vi "Dispense FN - OFF - Timer (SubVI).vi"(0 "Settings":T1={"ON Settings"={"Enable Dynamic Setpoint?"=TRUE, "Enable Dynamic Dispense Time?"=TRUE, "Enable Drain Rate Functions"=TRUE, "Dispense Sample Time (s)"=0.1, "Mass Average Samples"=20, "ON Timeout (sec)"=300.0, "1st Setpoint (% of Target)"=90.0, "2nd Setpoint (% of Target)"=95.0, "3rd Setpoint (% of Target)"=100.0, "Measure Dispense Delay (sec)"=10.0, "Minimum Spray Time (s)"=2.0, "Pump Reverse Time (s)"=10.0}, "OFF Settings"={"Drain Sample Time (s)"=0.1, "Drain Rate Ave Size"=100, "Drain Rate Limits (± g/sec)"=100.0, "Level Slope Range (± g/sec)"=0.05, "OFF Timeout (sec)"=300.0, "Near SP Slope Level (± g/sec)"=0.005, "Near Setpoint Threshold (%)"=99.0}, "Overshoot Settings"={"Time Limit (s)"=30.0, "Container MAX (g)"=1500.0, "Max FILL Slope (+/- g/sec)"=100.0, "% Overshot to Enable (>)"=3.0}, "FILL Timeout (s)"=300.0, "Full \nSettle Time (s)"=30.0, "Pre-Hydrate \nSpray Time (s)"=0.0, "Pre-Hydrate \nWait Time (s)"=10.0, "m Value "=1.0, "b Value"=0.0, "Enable Overshoot Adjust?"=FALSE} {"ON Settings"."Pump Reverse Time (s)" min=0.0 max=60.0; "OFF Settings"."Near SP Slope Level (± g/sec)" format="%.3g"; "OFF Settings"."Level Slope Range (± g/sec)" format="%.3g"}, 5 "Reset":bool) -> (14 "Sample":bool, 16 "Max Drain Complete?":bool, 19 "Elapsed Time (s)":dbl)   [LabVIEW 2011]
panel:
  # "ONLY ADJUST\nBOLD VALUES!"
  # "Corrected Mass = SDC Mass * m + b"
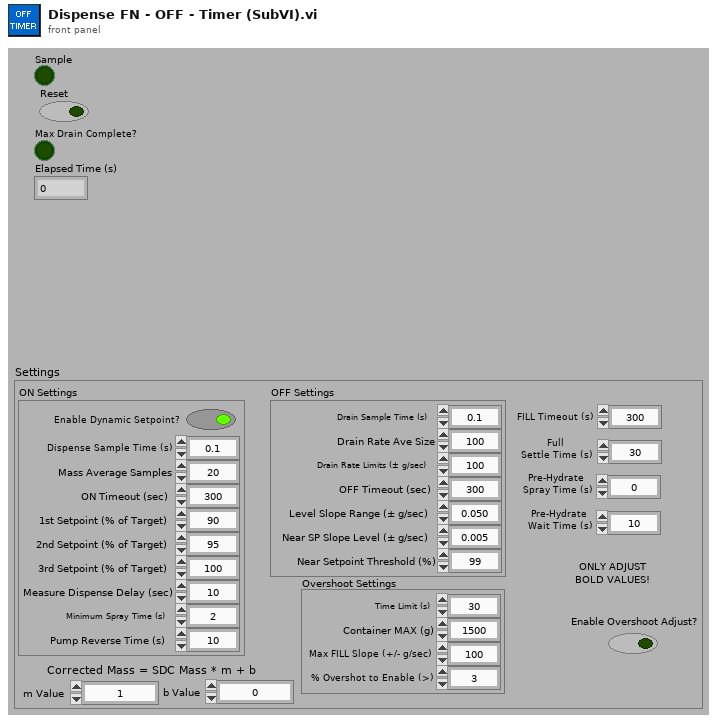
[diagram p1: front panel]
types:
  T1 = cluster{"ON Settings":cluster{"Enable Dynamic Setpoint?":bool, "Enable Dynamic Dispense Time?":bool, "Enable Drain Rate Functions":bool, "Dispense Sample Time (s)":dbl, "Mass Average Samples":i32, "ON Timeout (sec)":dbl, "1st Setpoint (% of Target)":dbl, "2nd Setpoint (% of Target)":dbl, "3rd Setpoint (% of Target)":dbl, "Measure Dispense Delay (sec)":dbl, "Minimum Spray Time (s)":dbl, "Pump Reverse Time (s)":dbl}, "OFF Settings":cluster{"Drain Sample Time (s)":dbl, "Drain Rate Ave Size":i32, "Drain Rate Limits (± g/sec)":dbl, "Level Slope Range (± g/sec)":dbl, "OFF Timeout (sec)":dbl, "Near SP Slope Level (± g/sec)":dbl, "Near Setpoint Threshold (%)":dbl}, "Overshoot Settings":cluster{"Time Limit (s)":dbl, "Container MAX (g)":dbl, "Max FILL Slope (+/- g/sec)":dbl, "% Overshot to Enable (>)":dbl}, "FILL Timeout (s)":dbl, "Full \nSettle Time (s)":dbl, "Pre-Hydrate \nSpray Time (s)":dbl, "Pre-Hydrate \nWait Time (s)":dbl, "m Value ":dbl, "b Value":dbl, "Enable Overshoot Adjust?":bool}
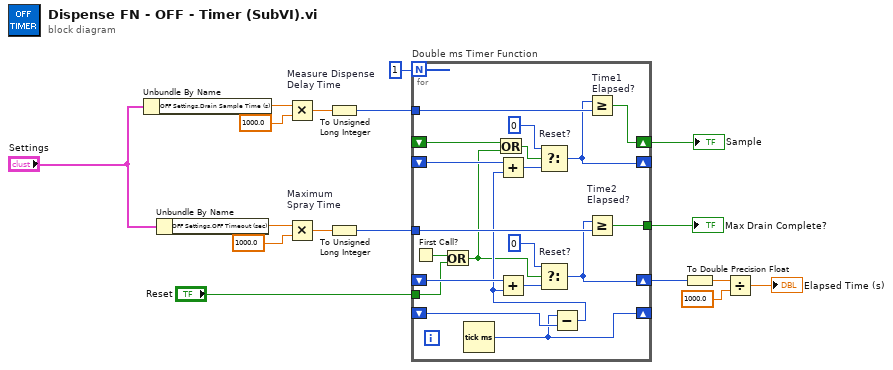
[diagram p0: block diagram]
diagram:
  n1 = Unbundle By Name("Settings") -> ("OFF Settings.Drain Sample Time (s)"=w14:dbl)
  n2 = Unbundle By Name("Settings") -> ("OFF Settings.OFF Timeout (sec)"=w13:dbl)
  n3 = Multiply "Measure Dispense\nDelay Time"(x=w14, y=1000.0) -> (x*y=w9:dbl)
  n4 = Multiply "Maximum\nSpray Time"(x=w13, y=1000.0) -> (x*y=w6:dbl)
  n5 = To Unsigned Long Integer(number=w9) -> (unsigned 32bit integer=w8:u32)
  n6 = To Unsigned Long Integer(number=w6) -> (unsigned 32bit integer=w5:u32)
  n7 = for "Double ms Timer Function" {
    N: 1 -> [_]
    shift-right: [w36] -> _
    shift-left: _ -> [w37]
    tunnel: w8 -> [w34]
    shift-right: [w28] -> w3
    shift-left: _ -> [w31]
    tunnel: w5 -> [w30]
    tunnel: [w29] -> w16
    tunnel: "Reset" -> [w26]
    shift-right: [w18] -> _
    shift-left: _ -> [w22]
    shift-right: [w35] -> w15
    shift-left: _ -> [w19]
    n8 = First Call?() -> (First Call?: T/F=w27:bool)
    n9 = Or(x=w27, y=w26) -> (x .or. y?=w21:bool)
    n10 = Tick Count (ms)() -> (millisecond timer value=w36:u32)
    n11 = Or(x=w19, y=w21) -> (x .or. y?=w20:bool)
    n12 = Subtract(x=w36, y=w37) -> (x-y=w23:u32)
    n13 = Add(x=w22, y=w23) -> (x+y=w25:u32)
    n14 = Add(x=w31, y=w23) -> (x+y=w33:u32)
    n15 = Select "Reset?"(t=u32 0, s=w20, f=w25) -> (s? t:f=w18:u32)
    n16 = Select "Reset?"(t=u32 0, s=w21, f=w33) -> (s? t:f=w28:u32)
    n17 = Greater Or Equal? "Time1\nElapsed?"(x=w18, y=w34) -> (x >= y?=w35:bool)
    n18 = Greater Or Equal? "Time2\nElapsed?"(x=w28, y=w30) -> (x >= y?=w29:bool)
  }
  "Max Drain Complete?" <- w16
  "Sample" <- w15
  n19 = To Double Precision Float(number=w3) -> (double precision float=w4:dbl)
  n20 = Divide(x=w4, y=1000.0) -> (x/y=→"Elapsed Time (s)":dbl)
